vi "Global Data.vi"() -> ()   [LabVIEW 2019]
panel:
  in  "Balls In Hopper":dbl
  out "LL Valid Targets?":bool
  in  "Climber Up Pos":dbl
  in  "Shooter Pos Max":dbl
  in  "Turret New Side Pos":dbl
  out "Turret Side Swap":bool
  in  "Turret Rotation Max":dbl
  in  "LL Angle Range (deg)":dbl=2.0
  in  "Idle Light":dbl=0.53
  in  "Nothing Light":dbl=0.61
  in  "Intake Down Light":dbl=0.69
  in  "Shooter Good Light":dbl=0.77
  out "MP Loaded":bool
  in  "LimeLight IP":string="10.43.43.11:5800"
  in  "Radius of Shooter (in)":dbl
  in  "Tick per Inch (angle)":dbl
  in  "Limelight TX":dbl
  in  "Target Center Height":dbl
  in  "Ball Release Height":dbl
  in  "Distance To Target (m)":dbl
  in  "Turret Tick Per Degree":dbl
  in  "Shooter Target Velocity":dbl
  in  "Shooter Present Velocity":dbl
  in  "Auto Selection":string
  # "Reference for colour:"
  # "Yellow"
  # "Green"
  # "http://www.revrobotics.com/content/docs/REV-11-1105-UM.pdf"
  # "Red"
  # "Yellow Blue Chasing"
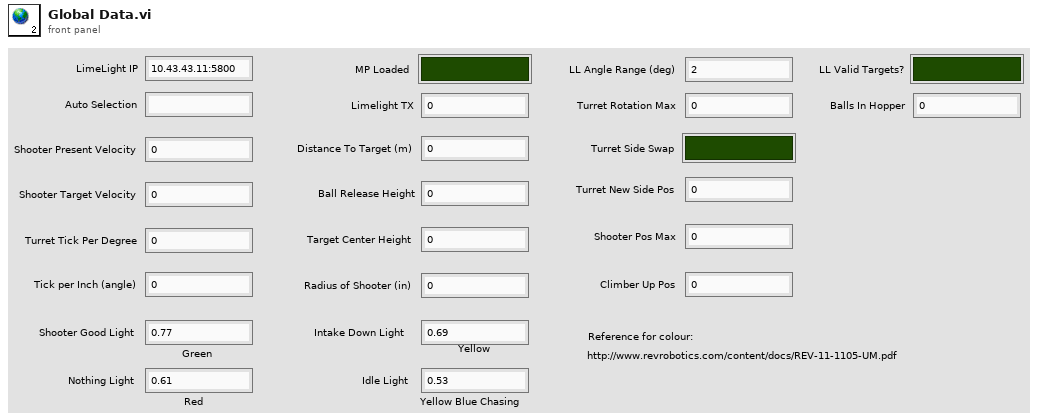
[diagram p1: front panel]
diagram:
